vi "Read end-stops -- subVI.vi"(8 "error in (no error)":errorcluster, 11 "VISA Refnum in":refnum<visa-resource-name>) -> (0 "error out":errorcluster, 3 "End-stops":cluster{"ES1":bool, "ES2":bool})   [LabVIEW 2020, in "Arduino stepper.lvlib"]
uses:
  Arduino stepper.lvlib
  <vilib>/Instr/_visa.llb/VISA Flush IO Buffer Mask.ctl
panel:
  out "read buffer":string
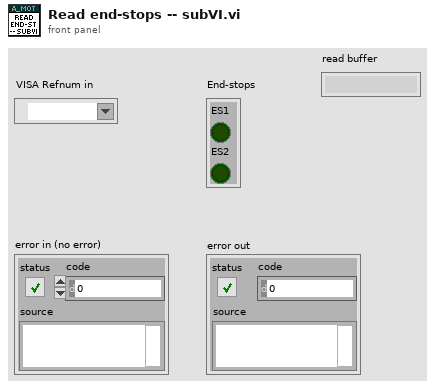
[diagram p1: front panel]
types:
  T1 = typedef "VISA Flush IO Buffer Mask.ctl" = u16
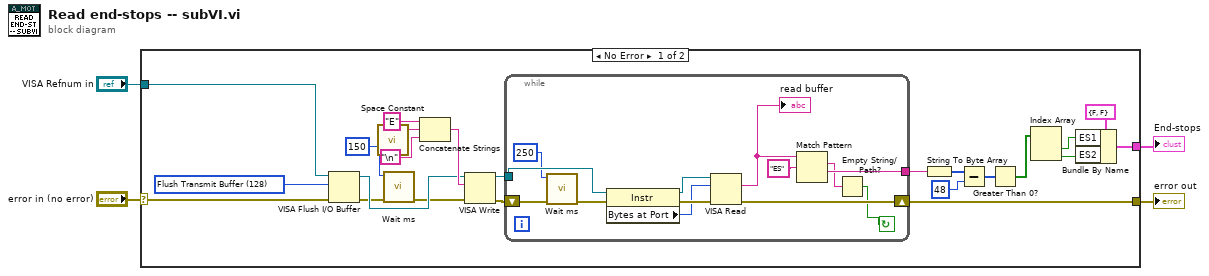
[diagram p0: block diagram]
diagram:
  n1 = case shown="No Error" "error in (no error)" {
    selector: "error in (no error)" -> [w18 w41]
    tunnel: [w16 w41] -> w4
    tunnel: "VISA Refnum in" -> [w20 _]
    tunnel: [w14 _] -> w1
    frame No Error {
      w6 = T1 128 items=["Flush Receive Buffer"=16, "Write Transmit Buffer to Device"=32, "Flush Receive Buffer (No I/O)"=64, "Flush Transmit Buffer"=128] ("Mask")
      n2 = VISA Flush I/O Buffer(VISA resource name=w20, mask (16)=w6, error in (no error)=w18) -> (VISA resource name out=w25:refnum<visa-resource-name>, error out=w19:errorcluster)
      n3 = call <vilib>:"Space Constant.vi"() -> ("String"=w5:string)
      n4 = call "Wait ms.vi"("error in (no error)"=w19, "milliseconds to wait"=u32 150) -> ("error out"=w24:errorcluster)  [unwired: 9 in]
      n5 = Concatenate Strings("E" ("string"), w5, "\n") -> (w26:string)
      n6 = VISA Write(VISA resource name=w25, write buffer=w26, error in (no error)=w24) -> (VISA resource name out=w17:refnum<visa-resource-name>, error out=w27:errorcluster)  [unwired: 1 out]
      n7 = while {
        tunnel: w17 -> [w39]
        tunnel: [w37] -> w13
        shift-right: [w38] -> w16
        shift-left: w27 -> [w40]
        stop <- w28 continue-if-true
        n8 = call "Wait ms.vi"("error in (no error)"=w40, "milliseconds to wait"=u32 250) -> ("error out"=w35:errorcluster)  [unwired: 9 in]
        n9 = property class="Instr"(reference=w39, error in=w35) -> (reference out=w33:refnum<visa-resource-name>, error out=w34:errorcluster, "Bytes at Port"=w32:u32)
        n10 = VISA Read(VISA resource name=w33, byte count=w32, error in (no error)=w34) -> (read buffer=w30:string, error out=w38:errorcluster)  [unwired: 2 out]
        "read buffer" <- w30
        n11 = Match Pattern(string=w30, regular expression="ES") -> (match substring=w29:string, after substring=w37:string)  [unwired: 1 in, 2 out]
        n12 = Empty String/Path?(string/path=w29) -> (empty?=w28:bool)
      }
      n13 = String To Byte Array(string=w13) -> (unsigned byte array=w12:u8[])
      n14 = Subtract(x=w12, y=u8 48) -> (x-y=w10:u8[])
      n15 = Greater Than 0?(x=w10) -> (x > 0?=w9:bool[])
      n16 = Index Array(array=w9) -> (element #1=w7:bool, element #2=w8:bool)  [unwired: 2 in]
      n17 = Bundle By Name(cluster=cluster{"ES1":bool, "ES2":bool} {"ES1"=FALSE, "ES2"=FALSE}, "ES1"=w7, "ES2"=w8) -> (w14:cluster{"ES1":bool, "ES2":bool})
    }
    frame Error {
    }
  }
  "error out" <- w4
  "End-stops" <- w1
